vi "Get Variables.vi"(8 "error in (no error)":errorcluster, 11 "For Loop in":refnum<class "While Loop.lvclass">) -> (0 "error out":errorcluster, 2 "Variables":variant, 3 "For Loop out":refnum<class "While Loop.lvclass">)   [LabVIEW 2016, in "While Loop.lvclass"]
uses:
  While Loop.lvclass
  While Loop.lvclass/While Loop.ctl
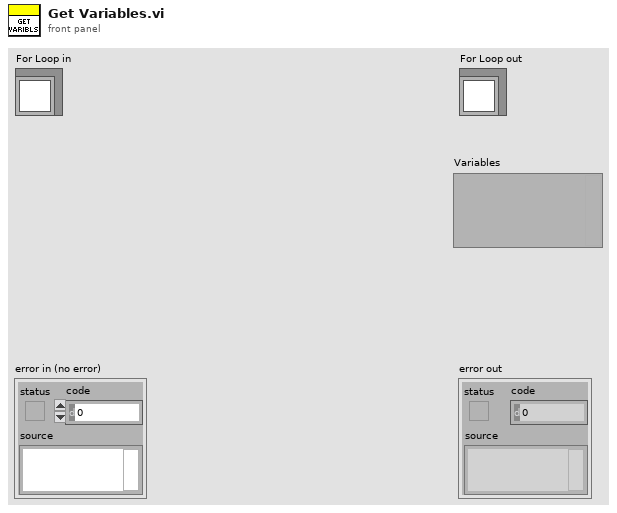
[diagram p1: front panel]
types:
  T1 = typedef "While Loop.lvclass/Variables.ctl" = cluster{"Continue?":bool}
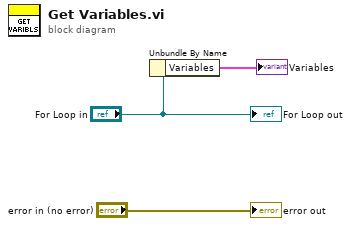
[diagram p0: block diagram]
diagram:
  n1 = Unbundle By Name("For Loop in") -> ("Variables"=→"Variables":T1)
  "error out" <- "error in (no error)"
  "For Loop out" <- "For Loop in"
